vi "Check Quick Editor.vi"(6 "Control Ref Queue":T1, 8 "error in (no error)":errorcluster, 9 "Array Element":refnum<vi>, 11 "Coords":T3) -> (0 "error out":errorcluster, 1 "Pop?":bool, 2 "Active Plot":i32, 3 "Window Bounds":T2)   [LabVIEW 2017, in "2D Plot.lvclass"]
uses:
  <vilib>/Math Plots/2D Math Plots/2D Plot/2D Plot/2D Plot.lvclass
  <vilib>/Utility/miscctls.llb/LVPoint32TypeDef.ctl
  <vilib>/Utility/miscctls.llb/LVRectTypeDef.ctl
  <vilib>/Math Plots/2D Math Plots/2D Plot/Action String/2DMathPlot Ctrl Act Queue.ctl
  <vilib>/Math Plots/2D Math Plots/2D Plot/Action String/2DMathPlot Ctrl Act Cluster.ctl
  <vilib>/Math Plots/2D Math Plots/2D Plot/Action String/2DMathPlot State Class.ctl
  <vilib>/Math Plots/Plot Private Lib/NI_Math Plot Private Lib.lvlib
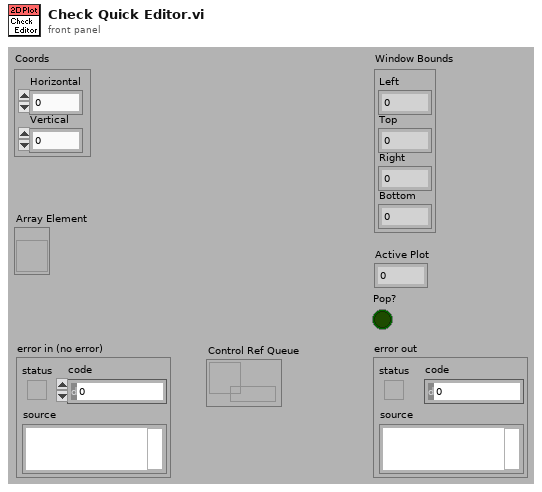
[diagram p1: front panel]
types:
  T1 = typedef "2DMathPlot Ctrl Act Queue.ctl" = refnum<queue>
  T2 = typedef "LVRectTypeDef.ctl" = cluster{"Left":i16, "Top":i16, "Right":i16, "Bottom":i16}
  T3 = typedef "LVPoint32TypeDef.ctl" = cluster{"Horizontal":i32, "Vertical":i32}
  T4 = typedef "2DMathPlot Ctrl Act Cluster.ctl" = cluster{"Plot Area Ref":refnum<vi>, "Z Axis Ref":refnum<vi>, "Legend Ref":refnum<vi>, "XControl Ref":refnum<vi>, "Facade Ref":refnum<vi>, "Display State Change Class":T5}
  T5 = typedef "2DMathPlot State Class.ctl" = enum16{"Update All (Undo)", "Update General", "Update Appearance", "Update Format", "Update Scale", "Update Marker", "Update Cursor", "None"}
  T6 = typedef "LVPositionTypeDef.ctl" = cluster{"Left":i32, "Top":i32}
  T7 = typedef "LVPointTypeDef.ctl" = cluster{"Horizontal":i16, "Vertical":i16}
  T8 = typedef "LVAllMonitorsDisplayTypeDef.ctl" = cluster{"Bounds":cluster{"Left":i16, "Top":i16, "Right":i16, "Bottom":i16}, "Depth":i16}[]
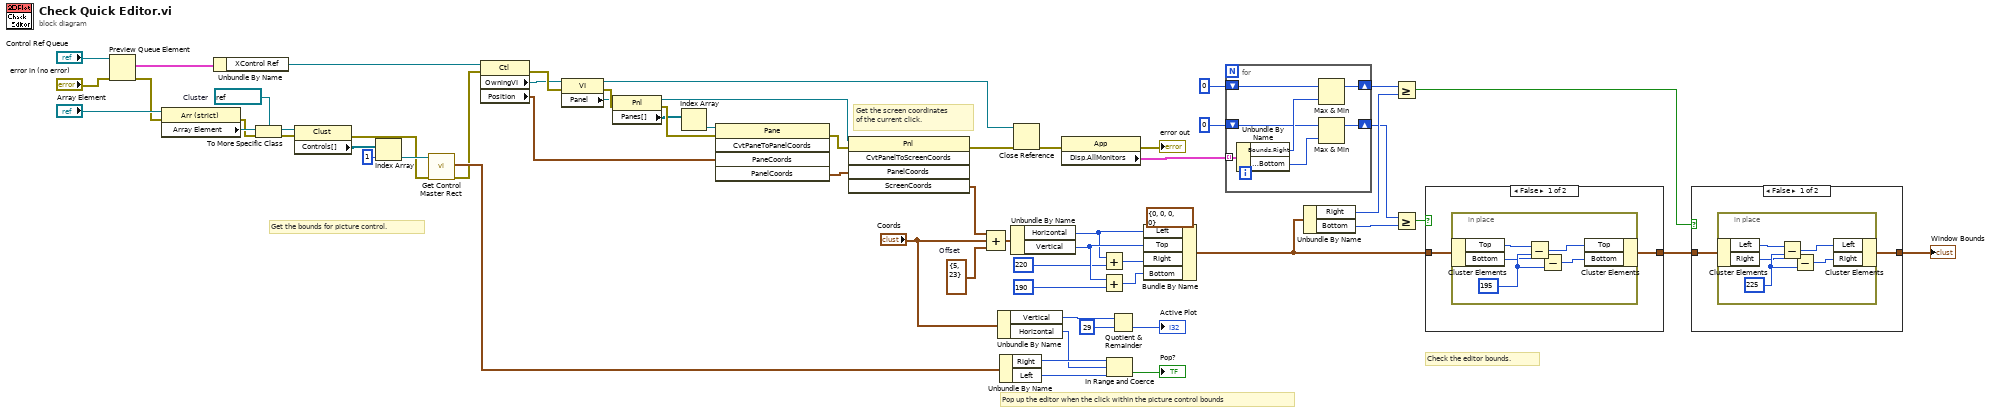
[diagram p0: block diagram]
diagram:
  w31 = refnum<vi> refnum  # Cluster
  w58 = T3 {"Horizontal"=5, "Vertical"=23}  # Offset
  # "Check the editor bounds."
  # "Get the screen coordinates\nof the current click."
  # "Get the bounds for picture control."
  # "Pop up the editor when the click within the picture control bounds"
  n1 = Preview Queue Element(queue="Control Ref Queue", error in (no error)="error in (no error)") -> (element=w35:T4, error out=w21:errorcluster)  [unwired: 3 out]
  n2 = property class="Arr (strict)"(reference="Array Element", error in=w21) -> (error out=w23:errorcluster, "Array Element"=w32:refnum<vi>)  [unwired: 1 out]
  n3 = Unbundle By Name(w35) -> ("XControl Ref"=w36:refnum<vi>)
  n4 = To More Specific Class(target class=w31, reference=w32, error in=w23) -> (specific class reference=w30:refnum<vi>, error out=w22:errorcluster)
  n5 = property class="Clust"(reference=w30, error in=w22) -> (error out=w18:errorcluster, "Controls[]"=w29:refnum<vi>[])  [unwired: 1 out]
  n6 = Index Array(array=w29, index=1) -> (element=w19:refnum<vi>)
  n7 = call <vilib>:"Get Control Master Rect.vi"("error in (no error)"=w18, "reference"=w19) -> ("error out"=w17:errorcluster, "Master Bounds Rect"=w20:T2)  [unwired: 8 out]
  n8 = property class="Ctl"(reference=w36, error in=w17) -> (error out=w54:errorcluster, "OwningVI"=w49:refnum<vi>, "Position"=w51:T6)  [unwired: 1 out]
  n9 = property class="VI"(reference=w49, error in=w54) -> (reference out=w16:refnum<vi>, error out=w55:errorcluster, "Panel"=w50:refnum<vi>)
  n10 = property class="Pnl"(reference=w50, error in=w55) -> (reference out=w46:refnum<vi>, error out=w56:errorcluster, "Panes[]"=w48:refnum<vi>[])
  n11 = Index Array(array=w48) -> (element=w47:refnum<vi>)  [unwired: 1 in]
  n12 = invoke class="Pane" method="CvtPaneToPanelCoords"(reference=w47, error in=w56, "PaneCoords"=w51) -> (error out=w57:errorcluster, "PanelCoords"=w52:T7)  [unwired: 2 in, 3 out]
  n13 = invoke class="Pnl" method="CvtPanelToScreenCoords"(reference=w46, error in=w57, "PanelCoords"=w52) -> (error out=w15:errorcluster, "ScreenCoords"=w53:T7)  [unwired: 2 in, 3 out]
  n14 = Compound Arithmetic op=ADD(w53, "Coords", w58) -> (w45:T3)
  n15 = Unbundle By Name("Coords") -> ("Vertical"=w60:i32, "Horizontal"=w25:i32)
  n16 = Unbundle By Name(w20) -> ("Right"=w27:i16, "Left"=w26:i16)
  n17 = Unbundle By Name(w45) -> ("Horizontal"=w39:i32, "Vertical"=w42:i32)
  n18 = Close Reference(reference=w16, error in (no error)=w15) -> (error out=w6:errorcluster)
  n19 = property class="App"(error in=w6) -> (error out=→"error out":errorcluster, "Disp.AllMonitors"=w14:T8)  [unwired: 1 in, 1 out]
  n20 = Add(x=w39, y=220) -> (x+y=w41:i32)
  n21 = Add(x=w42, y=190) -> (x+y=w43:i32)
  n22 = In Range and Coerce(upper limit=w27, x=w25, lower limit=w26) -> (In Range?=→"Pop?":bool)  [unwired: 1 out]
  n23 = Quotient & Remainder(x=w60, y=29) -> (floor(x/y)=→"Active Plot":i32)  [unwired: 1 out]
  n24 = Bundle By Name(cluster=T2 {"Left"=0, "Top"=0, "Right"=0, "Bottom"=0} ("Front Panel Window:Window Bounds"), "Left"=w39, "Top"=w42, "Right"=w41, "Bottom"=w43) -> (w4:T2)
  n25 = for {
    tunnel: w14 -> [w67] mode=indexing
    shift-right: [w68] -> w10
    shift-left: i16 0 -> [w69]
    shift-right: [w65] -> w9
    shift-left: i16 0 -> [w64]
    n26 = Unbundle By Name(w67) -> ("Bounds.Right"=w66:i16, "Bounds.Bottom"=w63:i16)
    n27 = Max & Min(x=w69, y=w66) -> (max(x,y)=w68:i16)  [unwired: 1 out]
    n28 = Max & Min(x=w64, y=w63) -> (max(x,y)=w65:i16)  [unwired: 1 out]
  }
  n29 = Unbundle By Name(w4) -> ("Right"=w11:i16, "Bottom"=w8:i16)
  n30 = Greater Or Equal?(x=w10, y=w11) -> (x >= y?=w1:bool)
  n31 = Greater Or Equal?(x=w9, y=w8) -> (x >= y?=w7:bool)
  n32 = case shown="False" w7 {
    tunnel: [w70 w77] -> w3
    tunnel: w4 -> [w71 w77]
    frame False {
      n33 = in-place {
        w74 = i16 195 ("y")
        n34 = in-place-cluster #1(w71) -> ("Top"=w76:i16, "Bottom"=w73:i16)
        n35 = Subtract(x=w76, y=w74) -> (x-y=w75:i16)
        n36 = Subtract(x=w73, y=w74) -> (x-y=w72:i16)
        n37 = in-place-cluster #1("Top"=w75, "Bottom"=w72) -> (w70:T2)
      }
    }
    frame True {
    }
  }
  n38 = case shown="False" w1 {
    tunnel: w3 -> [w79 w85]
    tunnel: [w78 w85] -> w2
    frame False {
      n39 = in-place {
        w82 = i16 225 ("y")
        n40 = in-place-cluster #2(w79) -> ("Left"=w84:i16, "Right"=w81:i16)
        n41 = Subtract(x=w84, y=w82) -> (x-y=w83:i16)
        n42 = Subtract(x=w81, y=w82) -> (x-y=w80:i16)
        n43 = in-place-cluster #2("Left"=w83, "Right"=w80) -> (w78:T2)
      }
    }
    frame True {
    }
  }
  "Window Bounds" <- w2
